vi "Initialize.vi"(8 "error in (no error)":errorcluster, 11 "Osciloscopio in":refnum<class "Osciloscopio.lvclass">) -> (0 "error out":errorcluster, 3 "Osciloscopio out":refnum<class "Osciloscopio.lvclass">)   [LabVIEW 2020, in "Oscilloscope.lvlib" / "Osciloscopio.lvclass"]
uses:
  Osciloscopio.lvclass
  Osciloscopio.lvclass/Osciloscopio.ctl
  <instrlib>/Tektronix TDS 200 1000 2000 Series/Tektronix TDS 200 1000 2000 Series.lvlib
panel:
  in  "ID Query? (T: Yes)":bool=TRUE
  in  "Reset? (T: Yes)":bool=TRUE
  in  "Serial Configuration":T1={"Baud Rate"=9600, "Parity"=0, "Stop Bits"=10, "Flow Control"=2} {"Flow Control" items=["None", "XON/XOFF", "RTS/CTS", "XON/XOFF & RTS/CTS", "DTR/DSR", "XON/XOFF & DTR/DSR"]; "Stop Bits" items=["1.0"=10, "1.5"=15, "2.0"=20]; "Parity" items=["None", "Odd", "Even", "Mark", "Space"]; "Baud Rate" items=["300"=300, "600"=600, "1200"=1200, "2400"=2400, "4800"=4800, "9600"=9600, "19200"=19200]}
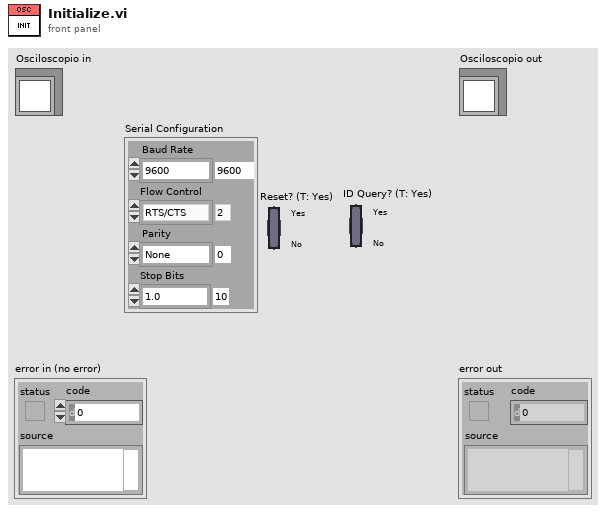
[diagram p1: front panel]
types:
  T1 = cluster{"Baud Rate":u32, "Parity":u16, "Stop Bits":u16, "Flow Control":u16}
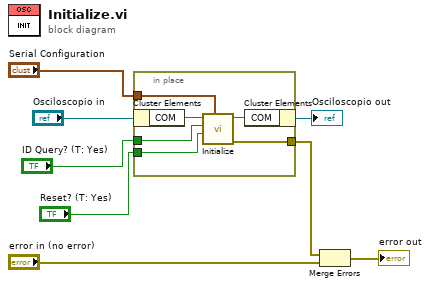
[diagram p0: block diagram]
diagram:
  n1 = in-place {
    in-place-border: "Serial Configuration" -> [w12]
    in-place-border: [w11] -> w1
    in-place-border: "ID Query? (T: Yes)" -> [w10]
    in-place-border: "Reset? (T: Yes)" -> [w9]
    n2 = in-place-cluster #1("Osciloscopio in") -> ("COM"=w13:refnum<visa-resource-name>)
    n3 = call <instrlib>:"Initialize.vi"("Serial Configuration"=w12, "Reset? (T: Yes)"=w9, "ID Query? (T: Yes)"=w10, "VISA resource name"=w13) -> ("error out"=w11:errorcluster, "VISA resource name out"=w14:refnum<visa-resource-name>)  [unwired: 6 in]
    n4 = in-place-cluster #1("COM"=w14) -> (→"Osciloscopio out":refnum<class "Osciloscopio.lvclass">)
  }
  n5 = Merge Errors(w1, "error in (no error)") -> (→"error out":errorcluster)
